vi "mod_op.vi"() -> ()   [LabVIEW 2019]
panel:
  out "Q":dbl
  out "R":dbl
  in  "Y":dbl
  in  "X":dbl
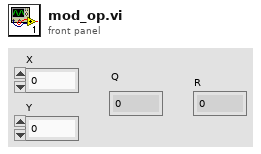
[diagram p1: front panel]
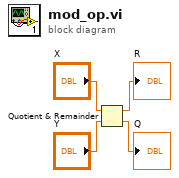
[diagram p0: block diagram]
diagram:
  n1 = Quotient & Remainder(x="X", y="Y") -> (x-y*floor(x/y)=→"R":dbl, floor(x/y)=→"Q":dbl)
